vi "Function.vi"(8 "error in (no error)":errorcluster, 9 "Bool B":T1, 10 "Bool A":T1, 11 "AND in":refnum<class "AND_Bool_1D.lvclass">) -> (0 "error out":errorcluster, 2 "Result":T1, 3 "AND out":refnum<class "AND_Bool_1D.lvclass">)   [LabVIEW 2021, in "AND_Bool_1D.lvclass"]
uses:
  AND_Bool_1D.lvclass
  Type.ctl
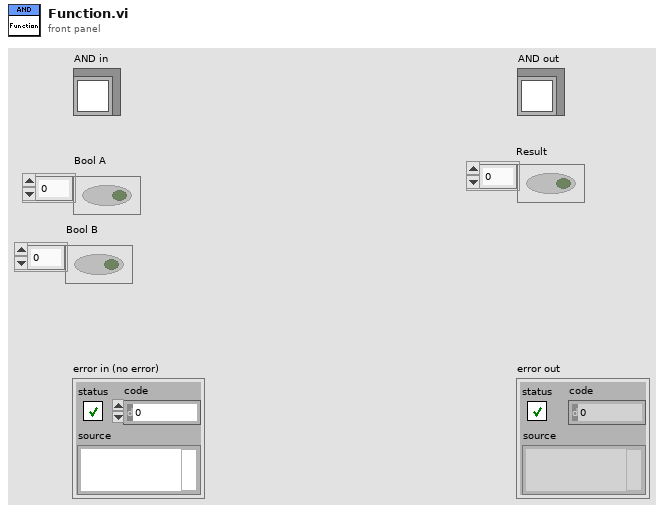
[diagram p1: front panel]
types:
  T1 = typedef "AND_Bool_1D.lvclass/Type.ctl" = bool[]
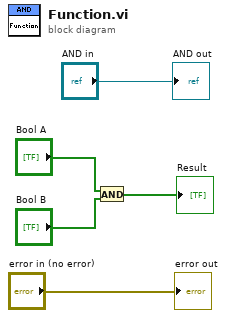
[diagram p0: block diagram]
diagram:
  n1 = And(x="Bool A", y="Bool B") -> (x .and. y?=→"Result":T1)
  "error out" <- "error in (no error)"
  "AND out" <- "AND in"
